vi "Conf Scan List.vi"(6 "Scan List (empty)":string, 8 "error in (no error)":errorcluster, 9 "Check Parameter (0:Scan List)":enum16{"Scan List", "Scan Size"}(ring), 10 "Set/Check (F:Set)":bool, 11 "VISA Resource Name":refnum<visa-resource-name>) -> (0 "error out":errorcluster, 2 "Configuration?":string, 3 "VISA Resource Name Out":refnum<visa-resource-name>)   [LabVIEW 2012, in "Agilent 34970.lvlib"]
doc: "This VI lets you configure or check the scan list.\n\nThis is an advanced configuration VI. For more information on the different ways to take and configure a measurment, refer to the context help and block diagram of \"HP34970A Advanced Scan Example.vi\"."
uses:
  <instrlib>/Agilent 34970/Agilent 34970.lvlib
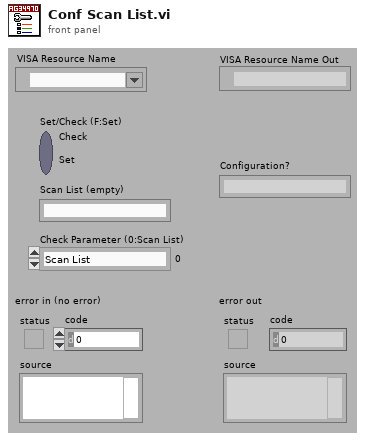
[diagram p1: front panel]
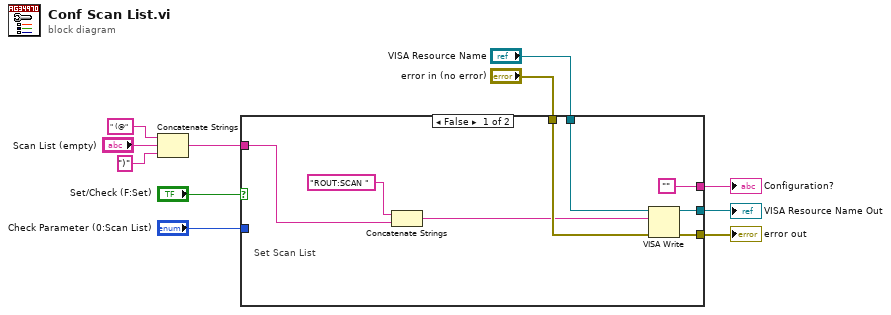
[diagram p0: block diagram]
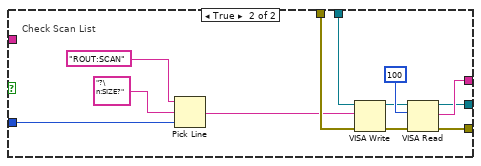
[diagram p2: hidden frame]
diagram:
  n1 = Concatenate Strings(" (@", "Scan List (empty)", ")") -> (w8:string)
  n2 = case shown="False" "Set/Check (F:Set)" {
    tunnel: [w15 w31] -> w3
    tunnel: [w16 w28] -> w4
    tunnel: w8 -> [w13 _]
    tunnel: ["" w29] -> w7
    tunnel: "VISA Resource Name" -> [w18 w27]
    tunnel: "error in (no error)" -> [w17 w26]
    tunnel: "Check Parameter (0:Scan List)" -> [_ w21]
    frame False {
      # "Set Scan List"
      n3 = Concatenate Strings("ROUT:SCAN ", w13) -> (w12:string)
      n4 = VISA Write(VISA resource name=w18, write buffer=w12, error in (no error)=w17) -> (VISA resource name out=w16:refnum<visa-resource-name>, error out=w15:errorcluster)  [unwired: 1 out]
    }
    frame True {
      # "Check Scan List"
      n5 = Pick Line(string ("")="ROUT:SCAN", multi-line string="?\n:SIZE?", line index=w21) -> (output string=w20:string)
      n6 = VISA Write(VISA resource name=w27, write buffer=w20, error in (no error)=w26) -> (VISA resource name out=w25:refnum<visa-resource-name>, error out=w24:errorcluster)  [unwired: 1 out]
      n7 = VISA Read(VISA resource name=w25, byte count=u32 100 ("byte count (0)"), error in (no error)=w24) -> (VISA resource name out=w28:refnum<visa-resource-name>, read buffer=w29:string, error out=w31:errorcluster)  [unwired: 1 out]
    }
  }
  "Configuration?" <- w7
  "VISA Resource Name Out" <- w4
  "error out" <- w3
